vi "Get Default Data From TD.vi"(8 "错误输入":errorcluster, 10 "Type Descriptor":T1) -> (0 "错误输出":errorcluster, 2 "Default VData":variant)   [LabVIEW 2012, in "TD Tools.lvlib"]
uses:
  TD Tools.lvlib
  Custom Type/Type Descriptor.ctl
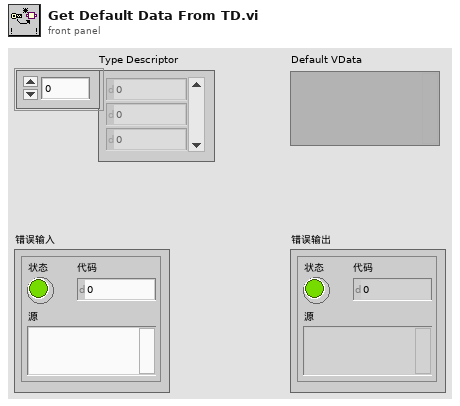
[diagram p1: front panel]
types:
  T1 = typedef "TD Tools.lvlib/Type Descriptor.ctl" = u16[]
  T2 = typedef "TD Tools.lvlib/Type Descriptor Header.ctl" = cluster{"length":u16, "private":u8, "type":T3, "# elements":u16}
  T3 = typedef "TD Tools.lvlib/Type Descriptor Enumeration.ctl" = enum16{"<Null>", "I8", "I16", "I32", "I64", "U8", "U16", "U32", "U64", "SGL", "DBL", "EXT", "CSG", "CDB", "CXT", "0x0F", "0x10", "0x11", "0x12", "0x13", "0x14", "Enum U8", "Enum U16", "Enum U32", "Enum U64", "SGL PQ", "DBL PQ", "EXT PQ", "CSG PQ", "CDB PQ", "CXT PQ", "0x1F", "0x20", "Boolean", "0x22", "0x23", "0x24", "0x25", "0x26", "0x27", "0x28", "0x29", "0x2A", "0x2B", "0x2C", "0x2D", "0x2E", "0x2F", "String", "0x31", "Path", "Pict", "0x34", "0x35", "0x36", "DAQ", "0x38", "0x39", "0x3A", "0x3B", "0x3C", "0x3D", "0x3E", "0x3F", "Array", "0x41", "0x42", "0x43", "0x44", "0x45", "0x46", "0x47", "0x48", "0x49", "0x4A", "0x4B", "0x4C", "0x4D", "0x4E", "0x4F", "Cluster", "0x51", "0x52", "Variant", "Waveform", "0x55", "0x56", "0x57", "0x58", "0x59", "0x5A", "0x5B", "0x5C", "0x5D", "0x5E", "0x5F", "0x60", "0x61", "0x62", "0x63", "0x64", "0x65", "0x66", "0x67", "0x68", "0x69", "0x6A", "0x6B", "0x6C", "0x6D", "0x6E", "0x6F", "Refnum"}
  T4 = typedef "Waveform Subtype Enum__ogtk.ctl" = enum8{"<Not a Waveform Type>", "0x01", "Analog 16-bit signed", "Analog Double-Precision", "0x04", "Analog Single Precision", "Timestamp", "Digital Data", "Digital Waveform", "Dynamic Data", "Analog Extended-Precision", "Analog 8-bit unsigned", "Analog 16-bit unsigned", "Analog 32-bit unsigned", "Analog 8-bit signed", "Analog 32-bit signed", "Analog Complex Single-Precision", "Analog Complex Double-Precision", "Analog Complex Extended Precision", "Analog 64-bit signed", "Analog 64-bit unsigned"}
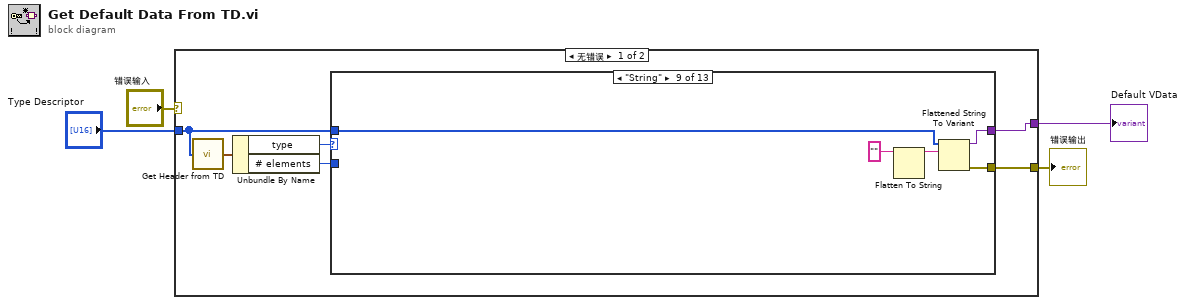
[diagram p0: block diagram]
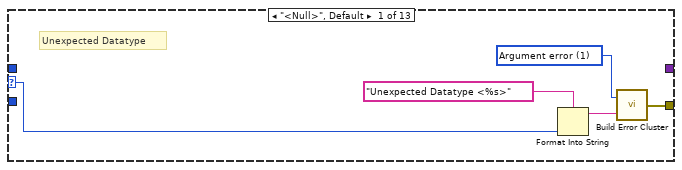
[diagram p2: hidden frame]
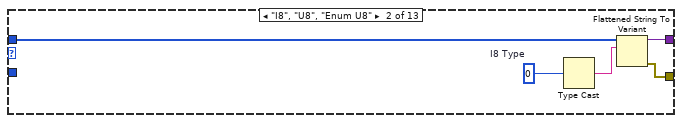
[diagram p3: hidden frame]
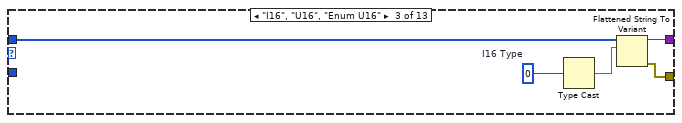
[diagram p4: hidden frame]
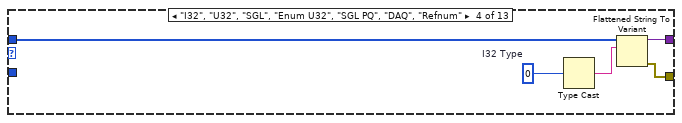
[diagram p5: hidden frame]
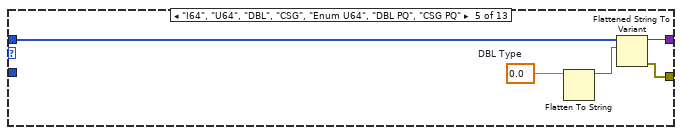
[diagram p6: hidden frame]
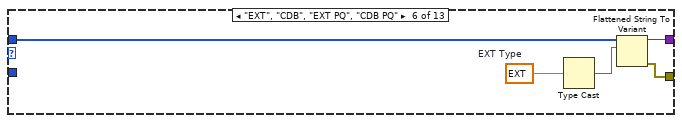
[diagram p7: hidden frame]
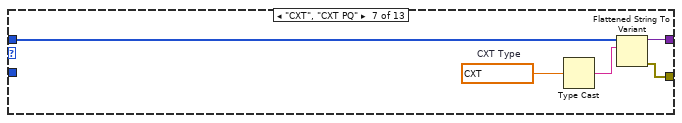
[diagram p8: hidden frame]
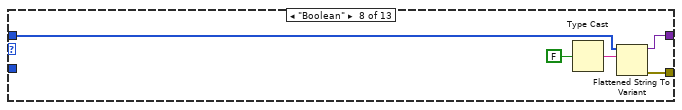
[diagram p9: hidden frame]
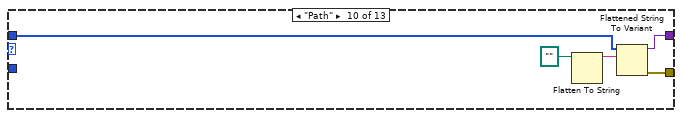
[diagram p10: hidden frame]
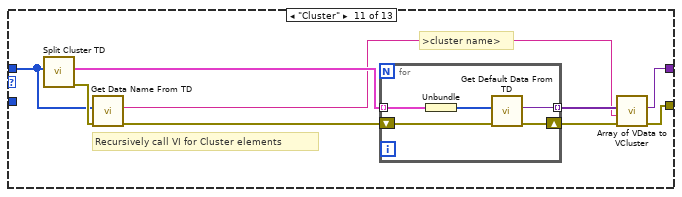
[diagram p11: hidden frame]
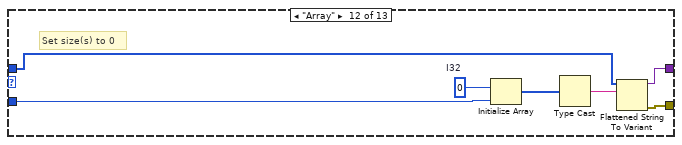
[diagram p12: hidden frame]
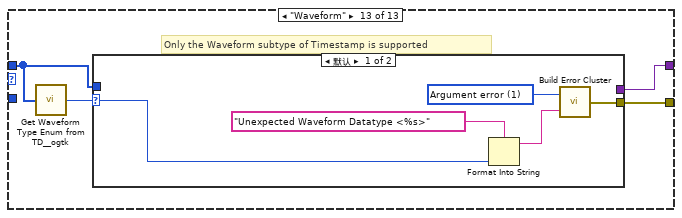
[diagram p13: hidden frame]
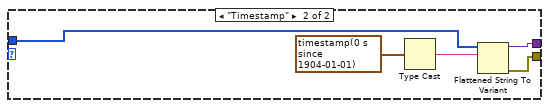
[diagram p14: hidden frame]
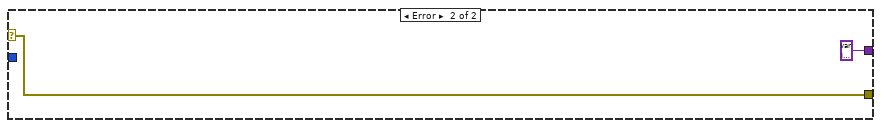
[diagram p15: hidden frame]
diagram:
  n1 = case shown="无错误" "错误输入" {
    selector: "错误输入" -> [_ w97]
    tunnel: [w10 w97] -> w1
    tunnel: "Type Descriptor" -> [w5 _]
    tunnel: [w9 variant] -> w2
    frame No Error {
      n2 = call "Get Header from TD.vi"("Type Desciptor"=w5) -> ("Type Descriptor Header"=w8:T2)
      n3 = Unbundle By Name(w8) -> ("type"=w7:T3, "# elements"=w6:u16)
      n4 = case shown="\"String\"" w7 {
        selector: w7 -> [w12 _ _ _ _ _ _ _ _ _ _ _ _]
        tunnel: [w11 w16 w23 w26 w32 w37 w43 w48 w51 w56 w63 w80 w84] -> w10
        tunnel: w5 -> [_ w18 w24 w28 w33 w39 w42 w49 w53 w59 w61 w79 w83]
        tunnel: [_ w17 w22 w27 w31 w36 w41 w46 w52 w57 w64 w81 w85] -> w9
        tunnel: w6 -> [_ _ _ _ _ _ _ _ _ _ _ w75 _]
        frame "<Null>", Default {
          w13 = 1 items=["No error", "Argument error", "Memory is full", "Out of zone", "End of file", "File already open", "Generic file I/O error", "File not found", "File permission error", "Disk is full", "Duplicate path", "Too many files open", "System feature not enabled", "Resource file not found", "Cannot add resource", "Resource not found", "Image not found", "Image memory error", "Pen does not exist", "Config type invalid", "Config token not found", "Config parse error", "Config memory error", "Bad external code format", "Bad external code offset", "External code not present", "Null window", "Destroy window error", "Null menu", "Print aborted", "Bad print record", "Print driver error", "Windows error during printing", "Memory error during printing", "Print dialog error", "Generic print error", "Invalid device refnum", "Device not found", "Device parameter error", "Device unit error", "Cannot open device", "Device call aborted", "Generic error", "Cancelled by user", "Object ID too low", "Object ID too high", "Object not in heap", "Unknown heap", "Unknown object (invalid DefProc)", "Unknown object (DefProc not in table)", "Message out of range", "Invalid (null) method", "Unknown message", "Manager call not supported", "Bad address", "Network operation in progress", "Network operation timed out", "Connection is busy", "Network attribute not supported", "Network error", "Address in use", "System out of memory", "Connection aborted", "Connection refused", "Not connected", "Already connected", "Connection closed", "Initialization error (interapplication manager)", "Bad occurrence", "Wait on unbound occurrence handler", "Occurrence queue overflow", "Datalog type conflict", "Unused", "Unrecognized type (interapplication manager)", "Memory corrupt", "Failed to make temporary DLL", "Old CIN version", "Drag socket not found", "Failed to load drop-object", "Failed to register OLE object", "Failed to release OLE object", "Format specifier type mismatch", "Unknown format specifier", "Too few format specifiers", "Too many format specifiers", "Scan failed", "Newer CIN version", "Error converting to variant", "Runtime menu error", "Password tampered", "Variant attribute not found", "Incompatible variant data type", "Event data is not available", "Event Store is not present", "Occurrence is not found", "Event Queue is not created", "Event info is not available", "Refnum passed is NULL", "Error retrieving Class GUID", "Error retrieving CoClass GUID", "Error retrieving TypeLib GUID.", "Bad built application magic bytes.", "Specific driver is different from the specific driver associated with the Logical Name.", "There is no session opened to the class driver.", "Max Error", "MAX - Error with config objects", "MAX - Error loading configuration", "MAX - Group not supported"]
          # "Unexpected Datatype"
          n5 = Format Into String(format string="Unexpected Datatype <%s>" ("Format String"), w12) -> (resulting string=w15:string)  [unwired: 2 in, 1 out]
          n6 = call "Build Error Cluster.vi"("String to Prepend to source (\"\")"=w15, "code"=w13) -> ("error out"=w11:errorcluster)
        }
        frame "I8", "U8", "Enum U8" {
          w20 = i8 0  # I8 Type
          n7 = Type Cast(x=w20) -> (*(type *) &x=w19:string)  [unwired: 1 in]
          n8 = Flattened String To Variant(6:w19, 7:w18) -> (0:w16:errorcluster, 3:w17:variant)  [unwired: 1 in]
        }
        frame "I16", "U16", "Enum U16" {
          w25 = i16 0  # I16 Type
          n9 = Type Cast(x=w25) -> (*(type *) &x=w21:string)  [unwired: 1 in]
          n10 = Flattened String To Variant(6:w21, 7:w24) -> (0:w23:errorcluster, 3:w22:variant)  [unwired: 1 in]
        }
        frame "I32", "U32", "SGL", "Enum U32", "SGL PQ", "DAQ", "Refnum" {
          w30 = 0  # I32 Type
          n11 = Type Cast(x=w30) -> (*(type *) &x=w29:string)  [unwired: 1 in]
          n12 = Flattened String To Variant(6:w29, 7:w28) -> (0:w26:errorcluster, 3:w27:variant)  [unwired: 1 in]
        }
        frame "I64", "U64", "DBL", "CSG", "Enum U64", "DBL PQ", "CSG PQ" {
          w35 = 0.0  # DBL Type
          n13 = Flatten To String(anything=w35) -> (data string=w34:string)  [unwired: 3 in, 2 out]
          n14 = Flattened String To Variant(6:w34, 7:w33) -> (0:w32:errorcluster, 3:w31:variant)  [unwired: 1 in]
        }
        frame "EXT", "CDB", "EXT PQ", "CDB PQ" {
          w40 = ext 0.0  # EXT Type
          n15 = Type Cast(x=w40) -> (*(type *) &x=w38:string)  [unwired: 1 in]
          n16 = Flattened String To Variant(6:w38, 7:w39) -> (0:w37:errorcluster, 3:w36:variant)  [unwired: 1 in]
        }
        frame "CXT", "CXT PQ" {
          w45 = cxt 0.0+0.0i  # CXT Type
          n17 = Type Cast(x=w45) -> (*(type *) &x=w44:string)  [unwired: 1 in]
          n18 = Flattened String To Variant(6:w44, 7:w42) -> (0:w43:errorcluster, 3:w41:variant)  [unwired: 1 in]
        }
        frame "Boolean" {
          n19 = Type Cast(x=FALSE ("status")) -> (*(type *) &x=w47:string)  [unwired: 1 in]
          n20 = Flattened String To Variant(6:w47, 7:w49) -> (0:w48:errorcluster, 3:w46:variant)  [unwired: 1 in]
        }
        frame "String" {
          n21 = Flatten To String(anything="") -> (data string=w54:string)  [unwired: 3 in, 2 out]
          n22 = Flattened String To Variant(6:w54, 7:w53) -> (0:w51:errorcluster, 3:w52:variant)  [unwired: 1 in]
        }
        frame "Path" {
          n23 = Flatten To String(anything=path "") -> (data string=w58:string)  [unwired: 3 in, 2 out]
          n24 = Flattened String To Variant(6:w58, 7:w59) -> (0:w56:errorcluster, 3:w57:variant)  [unwired: 1 in]
        }
        frame "Cluster" {
          # "Recursively call VI for Cluster elements"
          # ">cluster name>"
          n25 = call "Split Cluster TD.vi"("Type Descriptor"=w61) -> ("error out"=w66:errorcluster, "Type Descriptors"=w68:cluster{T1}[])  [unwired: 8 in]
          n26 = call "Get Data Name From TD.vi"("错误输入"=w66, "Type Descriptor"=w61) -> ("错误输出"=w62:errorcluster, "Name"=w65:string)  [unwired: 8 in]
          n27 = for {
            tunnel: w68 -> [w74] mode=indexing
            shift-right: [w71] -> w67
            shift-left: w62 -> [w73]
            tunnel: [w70] -> w69 mode=indexing
            n28 = Unbundle(w74) -> (w72:T1)
            n29 = call "Get Default Data From TD.vi"("错误输入"=w73, "Type Descriptor"=w72) -> ("错误输出"=w71:errorcluster, "Default VData"=w70:variant)  [unwired: 8 in]
          }
          n30 = call "Array of VData to VCluster.vi"("error in (no error)"=w67, "Cluster Name"=w65, "Array"=w69) -> ("error out"=w63:errorcluster, "VCluster"=w64:variant)  [unwired: 7 in]
        }
        frame "Array" {
          w78 = 0  # I32
          # "Set size(s) to 0"
          n31 = Initialize Array(w78, w75) -> (w77:i32[])
          n32 = Type Cast(x=w77) -> (*(type *) &x=w76:string)  [unwired: 1 in]
          n33 = Flattened String To Variant(6:w76, 7:w79) -> (0:w80:errorcluster, 3:w81:variant)  [unwired: 1 in]
        }
        frame "Waveform" {
          # "Only the Waveform subtype of Timestamp is supported"
          n34 = call <userlib>:"Get Waveform Type Enum from TD__ogtk.vi"("Type Descriptor"=w83) -> ("Waveform Subtype Enum"=w82:T4)  [unwired: 4 in]
          n35 = case shown="默认" w82 {
            selector: w82 -> [w86 _]
            tunnel: [_ w95] -> w85
            tunnel: [w87 w94] -> w84
            tunnel: w83 -> [_ w92]
            frame Default {
              w88 = 1 items=["No error", "Argument error", "Memory is full", "Out of zone", "End of file", "File already open", "Generic file I/O error", "File not found", "File permission error", "Disk is full", "Duplicate path", "Too many files open", "System feature not enabled", "Resource file not found", "Cannot add resource", "Resource not found", "Image not found", "Image memory error", "Pen does not exist", "Config type invalid", "Config token not found", "Config parse error", "Config memory error", "Bad external code format", "Bad external code offset", "External code not present", "Null window", "Destroy window error", "Null menu", "Print aborted", "Bad print record", "Print driver error", "Windows error during printing", "Memory error during printing", "Print dialog error", "Generic print error", "Invalid device refnum", "Device not found", "Device parameter error", "Device unit error", "Cannot open device", "Device call aborted", "Generic error", "Cancelled by user", "Object ID too low", "Object ID too high", "Object not in heap", "Unknown heap", "Unknown object (invalid DefProc)", "Unknown object (DefProc not in table)", "Message out of range", "Invalid (null) method", "Unknown message", "Manager call not supported", "Bad address", "Network operation in progress", "Network operation timed out", "Connection is busy", "Network attribute not supported", "Network error", "Address in use", "System out of memory", "Connection aborted", "Connection refused", "Not connected", "Already connected", "Connection closed", "Initialization error (interapplication manager)", "Bad occurrence", "Wait on unbound occurrence handler", "Occurrence queue overflow", "Datalog type conflict", "Unused", "Unrecognized type (interapplication manager)", "Memory corrupt", "Failed to make temporary DLL", "Old CIN version", "Drag socket not found", "Failed to load drop-object", "Failed to register OLE object", "Failed to release OLE object", "Format specifier type mismatch", "Unknown format specifier", "Too few format specifiers", "Too many format specifiers", "Scan failed", "Newer CIN version", "Error converting to variant", "Runtime menu error", "Password tampered", "Variant attribute not found", "Incompatible variant data type", "Event data is not available", "Event Store is not present", "Occurrence is not found", "Event Queue is not created", "Event info is not available", "Refnum passed is NULL", "Error retrieving Class GUID", "Error retrieving CoClass GUID", "Error retrieving TypeLib GUID.", "Bad built application magic bytes.", "Specific driver is different from the specific driver associated with the Logical Name.", "There is no session opened to the class driver.", "Max Error", "MAX - Error with config objects", "MAX - Error loading configuration", "MAX - Group not supported"]
              n36 = Format Into String(format string="Unexpected Waveform Datatype <%s>" ("Format String"), w86) -> (resulting string=w90:string)  [unwired: 2 in, 1 out]
              n37 = call "Build Error Cluster.vi"("String to Prepend to source (\"\")"=w90, "code"=w88) -> ("error out"=w87:errorcluster)
            }
            frame "Timestamp" {
              n38 = Type Cast(x=timestamp(0 s since 1904-01-01) ("Time Stamp")) -> (*(type *) &x=w93:string)  [unwired: 1 in]
              n39 = Flattened String To Variant(6:w93, 7:w92) -> (0:w94:errorcluster, 3:w95:variant)  [unwired: 1 in]
            }
          }
        }
      }
    }
    frame Error {
    }
  }
  "Default VData" <- w2
  "错误输出" <- w1
